vi "parameterXML.vi"() -> ()   [LabVIEW 2009, in "run.lvlib"]
uses:
  run.lvlib
  <vilib>/xml/Close Reference(Node).vi
  <vilib>/xml/Load XML String.vi
  <vilib>/xml/NI_XML.lvlib
  Program Files/National Instruments/LabVIEW 2009/resource/objmgr/DOMUserDefRef.rc
panel:
  in  "search 2":string="@parameter"
  out "Parameter values":string[][](array[string])
  out "Parameter nodes":string[][](array[string])
  in  "xml":string="<?xml version=\"1.0\" encoding=\"UTF-8\"  standalone='yes'?>\n<dataPoint>\n  <info>\n    <script_comment></script_comment>\n  </info>\n  <event_list>\n    <event time=\"0.\" channel_name=\"MOT coil\">\n      <time parameter=\"p10\">0.</time>\n      <time_difference parameter=\"p11\">0.</time_difference>\n      <channel_name>MOT coil</channel_name>\n      <action>changeValue</action>\n      <newValue>mot_loading</newValue>\n      <stage>Initialise</stage>\n      <comment></comment>\n    </event>\n    <event time=\"1000000.\" channel_name=\"analog2\">\n      <time parameter=\"freq\">1000000.</time>\n      <time_difference parameter=\"fred\">1000000.</time_difference>\n      <channel_name>analog2</channel_name>\n      <action>changeValue</action>\n      <newValue>on</newValue>\n      <stage>Initialise</stage>\n      <comment></comment>\n    </event>\n    <event time=\"2000000.\" channel_name=\"Cooling_AOM\">\n      <time>2000000.</time>\n      <time_difference parameter=\"joe\">1000000.</time_difference>\n      <channel_name>Cooling_AOM</channel_name>\n      <action>rf</action>\n      <additional_data>\n        <frequency parameter=\"mouki\">85000.</frequency>\n        <phase>0.</phase>\n      </additional_data>\n      <newValue>cooling</newValue>\n      <stage>Initialise</stage>\n      <comment></comment>\n    </event>\n  </event_list>\n</dataPoint>"
  in  "search":string=".//*[@parameter]"
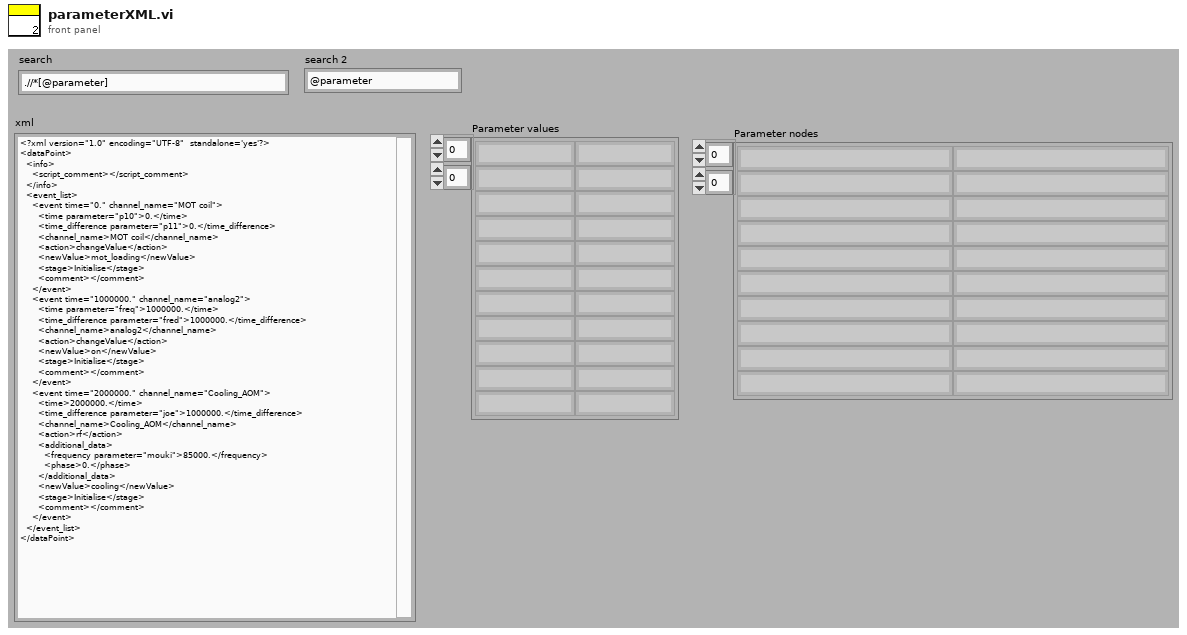
[diagram p1: front panel]
types:
  T1 = cluster{"parameter_name":string, "parameter_value":string, "type":enum16{"time", "time_difference", "value", "frequency", "phase", "ramp_time", "value_step", "time_step", "number_of_steps", "start_value", "end_value", "start_freq", "start_amp", "start_phase", "end_freq", "end_amp", "end_phase"}}
  T2 = enum16{"time", "time_difference", "value", "frequency", "phase", "ramp_time", "value_step", "time_step", "number_of_steps", "start_value", "end_value", "start_freq", "start_amp", "start_phase", "end_freq", "end_amp", "end_phase"}
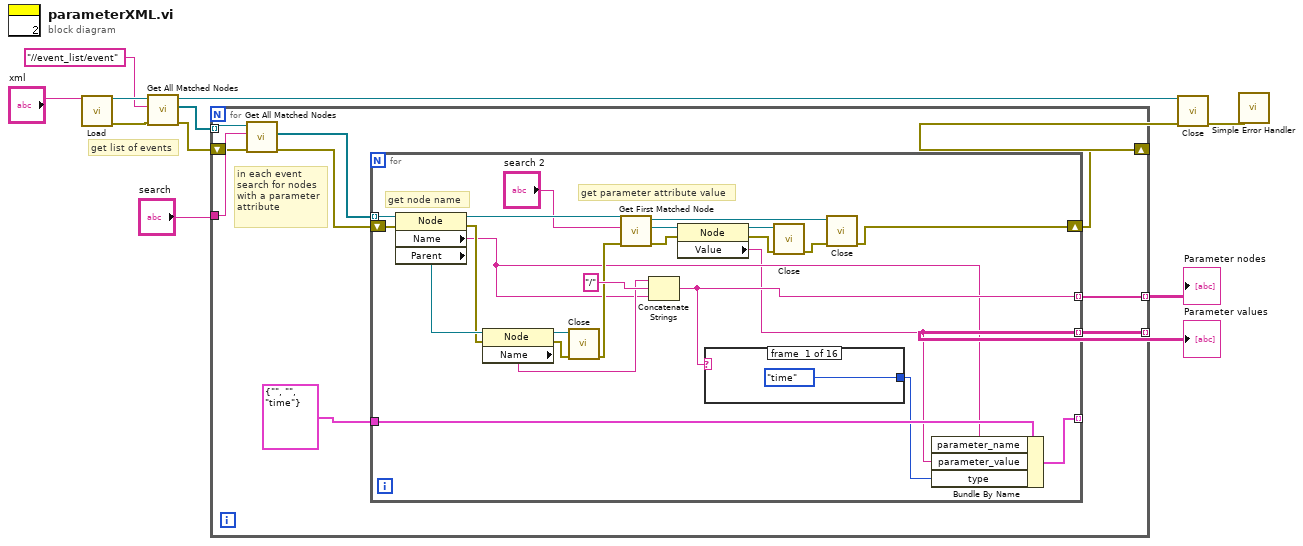
[diagram p0: block diagram]
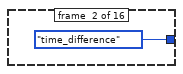
[diagram p2: hidden frame]
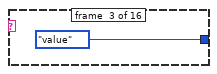
[diagram p3: hidden frame]
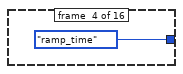
[diagram p4: hidden frame]
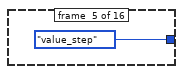
[diagram p5: hidden frame]
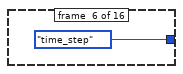
[diagram p6: hidden frame]
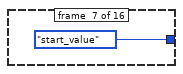
[diagram p7: hidden frame]
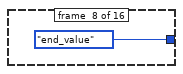
[diagram p8: hidden frame]
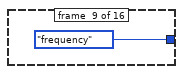
[diagram p9: hidden frame]
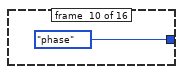
[diagram p10: hidden frame]
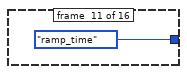
[diagram p11: hidden frame]
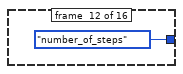
[diagram p12: hidden frame]
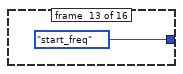
[diagram p13: hidden frame]
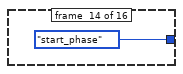
[diagram p14: hidden frame]
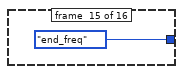
[diagram p15: hidden frame]
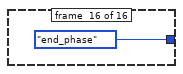
[diagram p16: hidden frame]
diagram:
  # "get list of events"
  n1 = call-poly <vilib>:"Load.vi"("XML string"="xml") -> ("DOM document out"=w10:refnum<k20>, "error out"=w9:errorcluster)  [unwired: 12 in, 1 out]
  n2 = call <vilib>:"Get All Matched Nodes.vi"("error in (no error)"=w9, "XPath expression"="//event_list/event", "node in"=w10) -> ("error out"=w1:errorcluster, "node result array"=w7:refnum<k20>[], "node out"=w6:refnum<k20>)  [unwired: 6 in]
  n3 = for {
    tunnel: "search" -> [w19]
    tunnel: w7 -> [w17] mode=indexing
    tunnel: [w16] -> w3 mode=indexing
    tunnel: [w15] -> w2 mode=indexing
    shift-right: [w18] -> w5
    shift-left: w1 -> [w14]
    # "in each event\nsearch for nodes\nwith a parameter\nattribute"
    n4 = call <vilib>:"Get All Matched Nodes.vi"("error in (no error)"=w14, "XPath expression"=w19, "node in"=w17) -> ("error out"=w20:errorcluster, "node result array"=w21:refnum<k20>[])  [unwired: 6 in, 1 out]
    n5 = for {
      tunnel: w21 -> [w45] mode=indexing
      shift-right: [w43] -> w18
      shift-left: w20 -> [w44]
      tunnel: [w27] -> w16 mode=indexing
      tunnel: [w24] -> w15 mode=indexing
      tunnel: T1 {"parameter_name"="", "parameter_value"="", "type"=enum."time"} ("param") -> [w26]
      tunnel: [w22] -> _ mode=indexing
      # "get parameter attribute value"
      # "get node name"
      n6 = property class="Node"(reference=w45, error in=w44) -> (reference out=w42:refnum<k20>, error out=w32:errorcluster, "Name"=w25:string, "Parent"=w33:refnum<k20>)
      n7 = property class="Node"(reference=w33, error in=w32) -> (reference out=w30:refnum<k20>, error out=w31:errorcluster, "Name"=w28:string)
      n8 = call-poly <vilib>:"Close.vi"("error in (no error)"=w31, "node"=w30) -> ("error out"=w29:errorcluster)  [unwired: 7 in]
      n9 = call <vilib>:"Get First Matched Node.vi"("error in (no error)"=w29, "XPath expression"="search 2", "node in"=w42) -> ("error out"=w39:errorcluster, "node result"=w40:refnum<k20>, "node out"=w35:refnum<k20>)  [unwired: 6 in]
      n10 = Concatenate Strings(w28, "/", w25) -> (w27:string)
      n11 = property class="Node"(reference=w40, error in=w39) -> (reference out=w38:refnum<k20>, error out=w37:errorcluster, "Value"=w24:string)
      n12 = case shown="\"stop/phase\"" w27 {
        tunnel: [T2."time" T2."time_difference" T2."value" T2."ramp_time" T2."value_step" T2."time_step" T2."start_value" T2."end_value" T2."frequency" T2."phase" T2."ramp_time" T2."number_of_steps" T2."start_freq" T2."start_phase" T2."end_freq" T2."end_phase"] -> w23
        frame #0 {
        }
        frame #1 {
        }
        frame #2 {
        }
        frame #3 {
        }
        frame #4 {
        }
        frame #5 {
        }
        frame #6 {
        }
        frame #7 {
        }
        frame #8 {
        }
        frame #9 {
        }
        frame #10 {
        }
        frame #11 {
        }
        frame #12 {
        }
        frame #13 {
        }
        frame #14 {
        }
        frame #15 {
        }
      }
      n13 = call-poly <vilib>:"Close.vi"("error in (no error)"=w37, "node"=w38) -> ("error out"=w36:errorcluster)  [unwired: 7 in]
      n14 = call-poly <vilib>:"Close.vi"("error in (no error)"=w36, "node"=w35) -> ("error out"=w43:errorcluster)  [unwired: 7 in]
      n15 = Bundle By Name(cluster=w26, "parameter_name"=w25, "parameter_value"=w24, "type"=w23) -> (w22:T1)
    }
  }
  "Parameter nodes" <- w3
  "Parameter values" <- w2
  n16 = call-poly <vilib>:"Close.vi"("error in (no error)"=w5, "node"=w6) -> ("error out"=w4:errorcluster)  [unwired: 7 in]
  n17 = call <vilib>:"Simple Error Handler.vi"("error in (no error)"=w4) -> ()  [unwired: 4 in, 5 out]
